vi "Construct ModelLogsAndClearsErrors.vi"() -> (1 "Final Error Notifier":refnum<notifier>, 3 "ModelLogsAndClearsErrors out":refnum<class "ModelLogsAndClearsErrors.lvclass">)   [LabVIEW 2017, in "ModelLogsAndClearsErrors.lvclass"]
uses:
  ModelLogsAndClearsErrors.lvclass
  ModelLogsAndClearsErrors.lvclass/ModelLogsAndClearsErrors.ctl
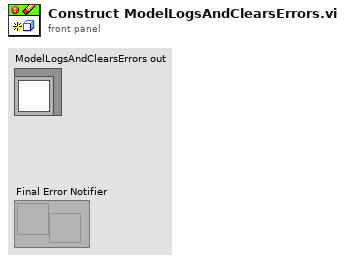
[diagram p1: front panel]
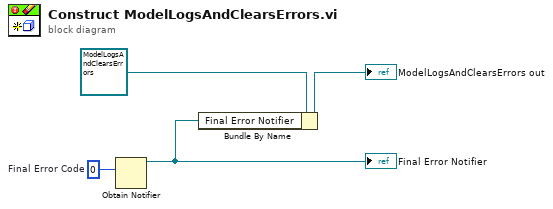
[diagram p0: block diagram]
diagram:
  w4 = 0  # Final Error Code
  n1 = Obtain Notifier(notification data type=w4) -> (notifier out=w3:refnum<notifier>)  [unwired: 3 in, 2 out]
  "Final Error Notifier" <- w3
  n2 = Bundle By Name(cluster=refnum<class "ModelLogsAndClearsErrors.lvclass"> refnum ("ModelLogsAndClearsErrors in"), "Final Error Notifier"=w3) -> (→"ModelLogsAndClearsErrors out":refnum<class "ModelLogsAndClearsErrors.lvclass">)
